vi "Configure Output Impedance.vi"(8 "error in (no error)":errorcluster, 9 "impedance (50 Ohms)":dbl[unit]=50.0 format="%.3f", 10 "channel name (\"CHANNEL1\")":string="CHANNEL1", 11 "CS++Fgen in":refnum<class "CS++Fgen.lvclass">) -> (0 "error out":errorcluster, 3 "CS++Fgen out":refnum<class "CS++Fgen.lvclass">)   [LabVIEW 2016, in "CS++Fgen.lvlib" / "CS++Fgen.lvclass"]
doc: "This VI configures the output impedance for the channel you specify."
uses:
  CS++Fgen.lvclass
  CSPP_Core/Classes/CS++ProcessVariables/ProcessVariable/PV.lvclass
  PV-Enum-n.ctl
  CSPP_Core/Classes/CS++ProcessVariables/ProcessVariable/PV.lvclass/PV.ctl
  CS++Fgen.lvclass/CS++Fgen.ctl
  CSPP_Core/Classes/CS++ProcessVariables/ProcessVariable/Write Data.vi
  CSPP_Core/Classes/CS++ProcessVariables/ProcessVariable/Write Timestamp.vi
  CSPP_Core/Classes/CS++ProcessVariables/ProcessVariable/Write Quality.vi
  CSPP_Core/Classes/CS++ProcessVariables/ProcessVariable/Write status.vi
  CSPP_Core/Classes/CS++ProcessVariables/PVConnection/PVConnection.lvclass
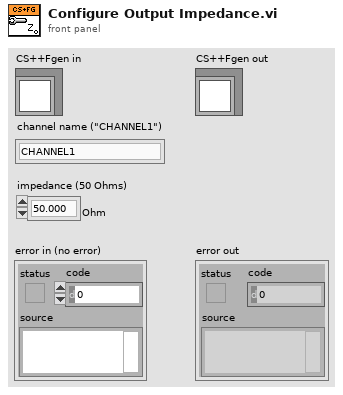
[diagram p1: front panel]
types:
  T1 = typedef "CS++Fgen.lvlib/CS++Fgen.lvclass/PV-Enum-n.ctl" = enum16{"Amplitude", "Arb-Frequency", "DCOffset", "Frequency", "OutputImpedance", "StartPhase", "AdvancedTriggerSlope", "AM-Source", "BurstCount", "FM-Source", "OperationMode", "ResumeTriggerSlope", "StartTriggerSlope", "StopTriggerSlope", "Waveform", "TriggerSource", "AM-Enabled", "ChannelEnabled", "FM-Enabled", "AdvancedTriggerSource", "ResumeTriggerSource", "StartTriggerSource", "StopTriggerSource"}
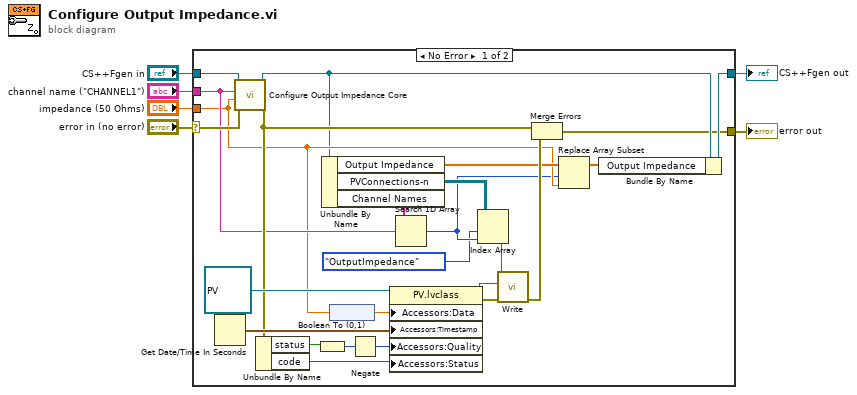
[diagram p0: block diagram]
diagram:
  n1 = case shown="No Error" "error in (no error)" {
    selector: "error in (no error)" -> [w30 w33]
    tunnel: [w10 w33] -> w5
    tunnel: [w11 w32] -> w3
    tunnel: "CS++Fgen in" -> [w31 w32]
    tunnel: "channel name (\"CHANNEL1\")" -> [w14 _]
    tunnel: "impedance (50 Ohms)" -> [w13 _]
    frame No Error {
      n2 = Get Date/Time In Seconds() -> (seconds since 1Jan1904=w29:timestamp)
      n3 = call-dynamic "Configure Output Impedance Core.vi"("error in (no error)"=w30, "impedance (50 Ohms)"=w13, "channel name (\"CHANNEL1\")"=w14, "CS++Fgen in"=w31) -> ("error out"=w15:errorcluster, "CS++Fgen out"=w12:refnum<class "CS++Fgen.lvclass">)  [unwired: 6 in]
      n4 = Unbundle By Name(w15) -> ("status"=w21:bool, "code"=w19:i32)
      n5 = Boolean To (0,1)(Boolean=w21) -> (0, 1=w20:i16)
      n6 = Unbundle By Name(w12) -> ("Output Impedance"=w17:dbl[unit][], "PVConnections-n"=w24:refnum<class "PVConnection.lvclass">[][], "Channel Names"=w25:string[])
      n7 = node(w13) -> (w9:dbl)
      n8 = Negate(x=w20) -> (-x=w18:i16)
      n9 = property class="PV.lvclass"(reference=refnum<class "PV.lvclass"> refnum ("PV"), "Accessors:Data"=w9, "Accessors:Timestamp"=w29, "Accessors:Quality"=w18, "Accessors:Status"=w19) -> (reference out=w26:refnum<class "PV.lvclass">, error out=w27:errorcluster)  [unwired: 1 in]
      n10 = Search 1D Array(1D array=w25, element=w14) -> (index of element=w8:i32)  [unwired: 1 in]
      n11 = Index Array(array=w24, index (row)=PV-Enum-n."OutputImpedance" ("PV-Enum-n"), index (col)=w8) -> (element=w23:refnum<class "PVConnection.lvclass">)
      n12 = call "Write.vi"("error in (no error)"=w27, "PV"=w26, "PVConnection in"=w23) -> ("error out"=w22:errorcluster)  [unwired: 7 in, 1 out]
      n13 = Merge Errors(w15, w22) -> (w10:errorcluster)
      n14 = Replace Array Subset(array=w17, new element=w13, index=w8) -> (w16:dbl[unit][])
      n15 = Bundle By Name(cluster=w12, "Output Impedance"=w16) -> (w11:refnum<class "CS++Fgen.lvclass">)
    }
    frame Error {
    }
  }
  "error out" <- w5
  "CS++Fgen out" <- w3
